vi "closeAllRefs.vi"(8 "error in (no error)":errorcluster, 11 "ImageStreamViewer in":refnum<class "ImageStreamViewer.lvclass">) -> (0 "error out":errorcluster, 3 "ImageStreamViewer out":refnum<class "ImageStreamViewer.lvclass">)   [LabVIEW 2009, in "Views.lvlib" / "Camera.lvlib" / "ImageStreamViewer.lvclass"]
uses:
  ImageStreamViewer.lvclass
  ImageStreamViewer.lvclass/ImageStreamViewer.ctl
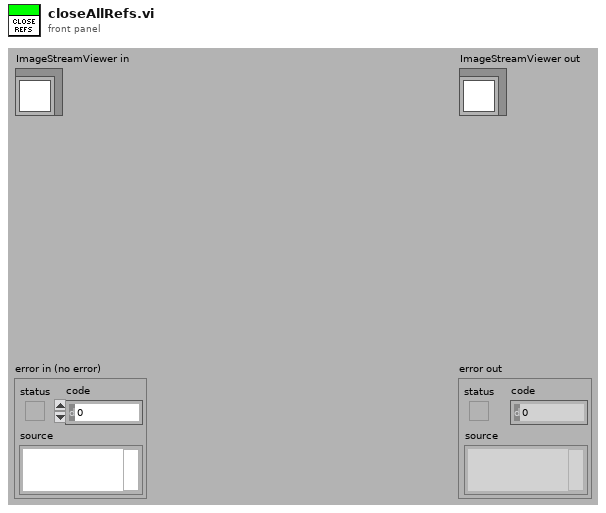
[diagram p1: front panel]
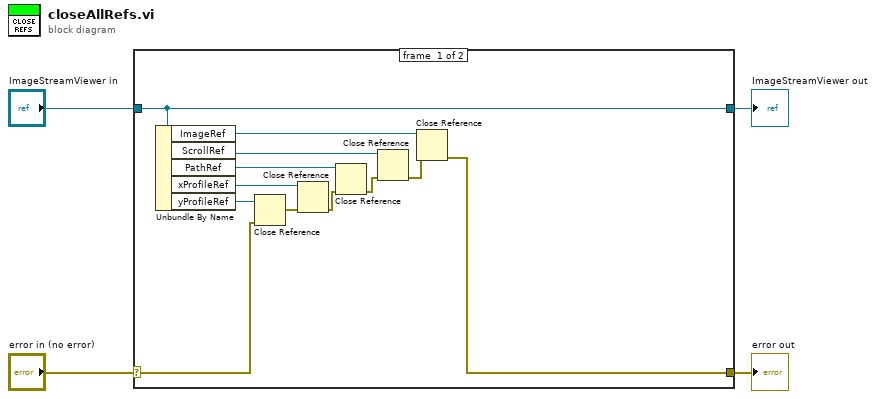
[diagram p0: block diagram]
diagram:
  n1 = case shown="No Error" "error in (no error)" {
    selector: "error in (no error)" -> [w6 w18]
    tunnel: [w5 w18] -> w3
    tunnel: [w16 w17] -> w1
    tunnel: "ImageStreamViewer in" -> [w16 w17]
    frame #0 {
      n2 = Unbundle By Name(w16) -> ("ImageRef"=w11:refnum<vi>, "ScrollRef"=w10:refnum<vi>, "PathRef"=w9:refnum<vi>, "xProfileRef"=w8:refnum<vi>, "yProfileRef"=w7:refnum<vi>)
      n3 = Close Reference(reference=w7, error in (no error)=w6) -> (error out=w15:errorcluster)
      n4 = Close Reference(reference=w8, error in (no error)=w15) -> (error out=w14:errorcluster)
      n5 = Close Reference(reference=w9, error in (no error)=w14) -> (error out=w13:errorcluster)
      n6 = Close Reference(reference=w10, error in (no error)=w13) -> (error out=w12:errorcluster)
      n7 = Close Reference(reference=w11, error in (no error)=w12) -> (error out=w5:errorcluster)
    }
    frame #1 {
    }
  }
  "error out" <- w3
  "ImageStreamViewer out" <- w1
